vi "CRYCheck dB ref unit.vi"(9 "dB ref in":dbl, 11 "Unit in":string) -> (0 "dB re":string, 1 "dB ref N/dB ref N **?":bool, 2 "Lin unit out":string, 3 "Unit out":string)   [LabVIEW 2013]
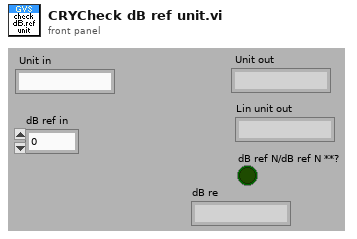
[diagram p1: front panel]
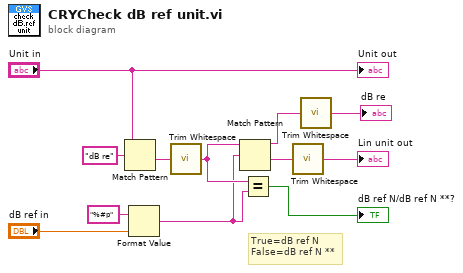
[diagram p0: block diagram]
diagram:
  # "True=dB ref N\nFalse=dB ref N **"
  n1 = Match Pattern(string="Unit in", regular expression="dB re") -> (after substring=w7:string)  [unwired: 4 out]
  n2 = Format Value(format string="%#p", value (0)="dB ref in") -> (output string=w5:string)  [unwired: 1 in]
  n3 = call <vilib>:"Trim Whitespace.vi"("string"=w7) -> ("trimmed string"=w6:string)  [unwired: 1 in]
  n4 = Match Pattern(string=w6, regular expression=w5) -> (before substring=w2:string, after substring=w4:string)  [unwired: 3 out]
  n5 = Equal?(x=w6, y=w5) -> (x = y?=→"dB ref N/dB ref N **?":bool)
  n6 = call <vilib>:"Trim Whitespace.vi"("string"=w4) -> ("trimmed string"=→"Lin unit out":string)  [unwired: 1 in]
  n7 = call <vilib>:"Trim Whitespace.vi"("string"=w2) -> ("trimmed string"=→"dB re":string)  [unwired: 1 in]
  "Unit out" <- "Unit in"
